vi "例6-10.vi"() -> ()   [LabVIEW 2019]
uses:
  <vilib>/Analysis/2dsp.llb/Real FFT.vi
  <vilib>/Analysis/NI_AALPro.lvlib
  <vilib>/Analysis/NI_AALBase.lvlib
panel:
  in  "采样点数":dbl=100.0
  in  "采样频率":dbl=100.0
  in  "幅值2":dbl=2.0
  in  "频率2":dbl=20.0
  in  "幅值1":dbl=1.0
  in  "频率1":dbl=10.0
  out "频域波形":cluster{dbl, dbl, dbl[]}(graph)
  out "时域波形":cluster{i32, dbl, dbl[]}(graph)
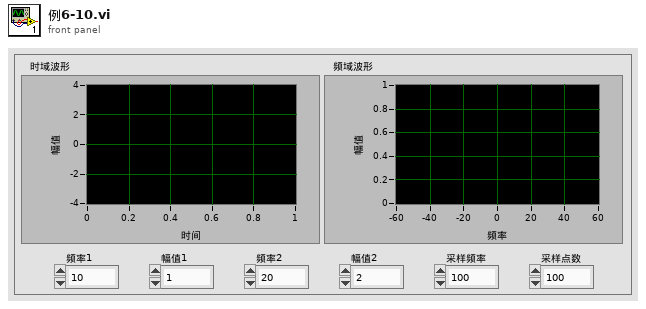
[diagram p1: front panel]
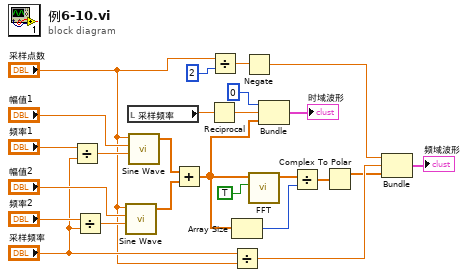
[diagram p0: block diagram]
diagram:
  n1 = Divide(x="频率1", y="采样频率") -> (x/y=w22:dbl)
  n2 = Divide(x="频率2", y="采样频率") -> (x/y=w23:dbl)
  n3 = call <vilib>:"Sine Wave.vi"("samples"="采样点数", "amplitude"="幅值2", "frequency"=w23) -> ("sine wave"=w18:dbl[])  [unwired: 2 in, 2 out]
  n4 = local read "采样频率"() -> (w16:dbl)
  n5 = call <vilib>:"Sine Wave.vi"("samples"="采样点数", "amplitude"="幅值1", "frequency"=w22) -> ("sine wave"=w19:dbl[])  [unwired: 2 in, 2 out]
  n6 = Add(x=w19, y=w18) -> (x+y=w13:dbl[])
  n7 = Reciprocal(x=w16) -> (1/x=w15:dbl)
  n8 = Divide(x="采样点数", y=2) -> (x/y=w3:dbl)
  n9 = Array Size(array=w13) -> (size(s)=w11:i32)
  n10 = Divide(x="采样频率", y="采样点数") -> (x/y=w8:dbl)
  n11 = Negate(x=w3) -> (-x=w2:dbl)
  n12 = call-poly <vilib>:"FFT.vi"("shift?"=TRUE, "X"=w13) -> ("FFT {X}"=w12:cdb[])  [unwired: 8 in, 1 out]
  n13 = Bundle(0, w15, w13) -> (→"时域波形":cluster{i32, dbl, dbl[]})  [unwired: 1 in]
  n14 = Divide(x=w12, y=w11) -> (x/y=w10:cdb[])
  n15 = Complex To Polar(r * e^(i*theta)=w10) -> (r=w7:dbl[])  [unwired: 1 out]
  n16 = Bundle(w2, w8, w7) -> (→"频域波形":cluster{dbl, dbl, dbl[]})  [unwired: 1 in]
